vi "Test Rename State.vi"(8 "error in (no error)":errorcluster) -> (0 "error out":errorcluster)   [LabVIEW 2013, in "JKI State Machine API - Tests.lvlib"]
uses:
  JKI State Machine API - Tests.lvlib
  source/JKI SM/JKI SM.lvclass
  <vilib>/addons/_JKI Toolkits/Caraya/classes/Test/Test.lvclass
  <vilib>/addons/_JKI Toolkits/Caraya/classes/Assert/Assert.lvclass
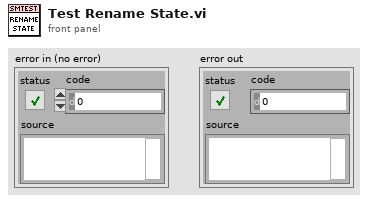
[diagram p1: front panel]
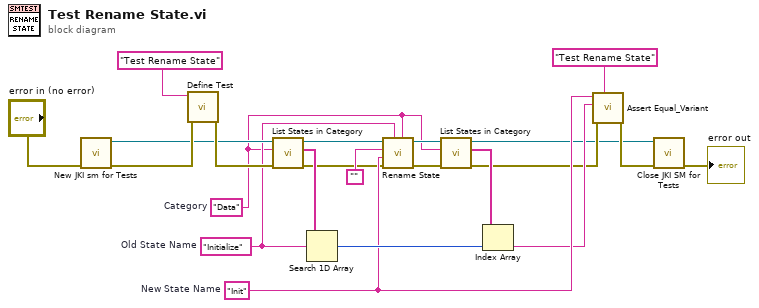
[diagram p0: block diagram]
diagram:
  w6 = "Init"  # New State Name
  w12 = "Initialize"  # Old State Name
  w9 = "Data"  # Category
  n1 = call "New JKI sm for Tests.vi"("error in (no error)"="error in (no error)") -> ("error out"=w16:errorcluster, "JKI SM out"=w15:refnum<class "JKI SM.lvclass">)  [unwired: 9 in]
  n2 = call <vilib>:"Define Test.vi"("error in (no error)"=w16, "Label (VI Title)"="Test Rename State") -> ("error out"=w22:errorcluster)  [unwired: 9 in]
  n3 = call "List States in Category.vi"("error in (no error)"=w22, "Category"=w9, "JKI SM in"=w15) -> ("error out"=w1:errorcluster, "States"=w14:string[], "JKI SM out"=w13:refnum<class "JKI SM.lvclass">)  [unwired: 4 in, 2 out]
  n4 = Search 1D Array(1D array=w14, element=w12) -> (index of element=w7:i32)  [unwired: 1 in]
  n5 = call-dynamic "Rename State.vi"("Category"=w9, "State"=w12, "error in (no error)"=w1, "New State"=w6, "New Category (\"\": Use Existing)"="" ("New Category (\"\": Use Existing)"), "JKI SM in"=w13) -> ("error out"=w11:errorcluster, "JKI SM out"=w10:refnum<class "JKI SM.lvclass">)  [unwired: 4 in]
  n6 = call "List States in Category.vi"("error in (no error)"=w11, "Category"=w9, "JKI SM in"=w10) -> ("error out"=w4:errorcluster, "States"=w8:string[], "JKI SM out"=w3:refnum<class "JKI SM.lvclass">)  [unwired: 4 in, 2 out]
  n7 = Index Array(array=w8, index=w7) -> (element=w5:string)
  n8 = call <vilib>:"Assert Equal_Variant.vi"("Label"="Test Rename State", "error in (no error)"=w4, "Y"=w5, "X"=w6) -> ("error out"=w19:errorcluster)  [unwired: 7 in]
  n9 = call "Close JKI SM for Tests.vi"("error in (no error)"=w19, "JKI SM in"=w3) -> ("error out"=→"error out":errorcluster)  [unwired: 9 in]
